vi "CheckStopCondition.vi"(5 "Lower limit":T1={"Fz [pN]"=-100000000.0, "Zext [nm]"=-100000000.0, "Tau [pNnm]"=-100000000.0, "Turn"=-100000000.0, "Fx [pN]"=-100000000.0, "Xext [nm]"=-100000000.0, "Fy [pN]"=-100000000.0, "Yext [nm]"=-100000000.0, "time [s]"=-100000000.0, "Delta Z signal"=-100000000.0, "Delta Z bead [nm]"=-100000000.0, "Z bead [nm]"=-100000000.0, "Delta TrapZ [nm]"=-100000000.0, "Delta Xsignal"=0.0, "X bead [nm]"=-100000000.0, "Delta Ysignal"=-100000000.0, "Y bead [nm]"=-100000000.0, "Stop Condition"=0.0}, 6 "Data":T1, 7 "Upper limit":T1={"Fz [pN]"=100000000.0, "Zext [nm]"=100000000.0, "Tau [pNnm]"=100000000.0, "Turn"=100000000.0, "Fx [pN]"=100000000.0, "Xext [nm]"=100000000.0, "Fy [pN]"=100000000.0, "Yext [nm]"=100000000.0, "time [s]"=100000000.0, "Delta Z signal"=100000000.0, "Delta Z bead [nm]"=100000000.0, "Z bead [nm]"=100000000.0, "Delta TrapZ [nm]"=100000000.0, "Delta Xsignal"=100000000.0, "X bead [nm]"=100000000.0, "Delta Ysignal"=100000000.0, "Y bead [nm]"=100000000.0, "Stop Condition"=100000000.0}) -> (1 "In range?":bool, 2 "Which Signal is out of Range?":u32, 3 "Data out":T1)   [LabVIEW 2020, in "SignalConverson.lvlib"]
uses:
  SignalConverson.lvlib
  Initialization/Physical Quantitites.ctl
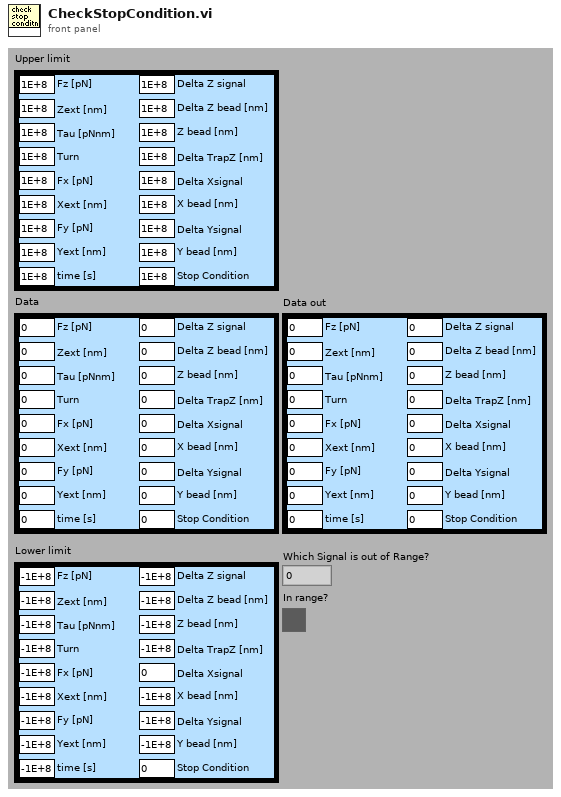
[diagram p1: front panel]
types:
  T1 = typedef "SignalConverson.lvlib/Physical Quantitites.ctl" = cluster{"Fz [pN]":dbl, "Zext [nm]":dbl, "Tau [pNnm]":dbl, "Turn":dbl, "Fx [pN]":dbl, "Xext [nm]":dbl, "Fy [pN]":dbl, "Yext [nm]":dbl, "time [s]":dbl, "Delta Z signal":dbl, "Delta Z bead [nm]":dbl, "Z bead [nm]":dbl, "Delta TrapZ [nm]":dbl, "Delta Xsignal":dbl, "X bead [nm]":dbl, "Delta Ysignal":dbl, "Y bead [nm]":dbl, "Stop Condition":dbl}
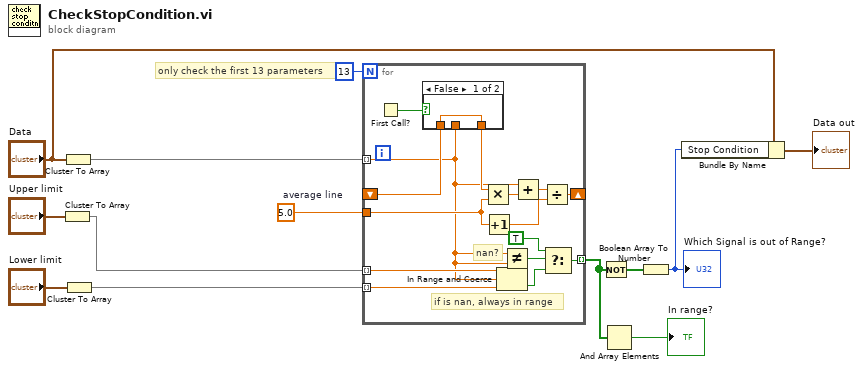
[diagram p0: block diagram]
diagram:
  w6 = 5.0  # average line
  # "only check the first 13 parameters"
  n1 = Cluster To Array(cluster="Upper limit") -> (array=w12:dbl[])
  n2 = Cluster To Array(cluster="Data") -> (array=w10:dbl[])
  n3 = Cluster To Array(cluster="Lower limit") -> (array=w11:dbl[])
  n4 = for {
    N: 13 -> [_]
    tunnel: w12 -> [w28] mode=indexing
    tunnel: w11 -> [w27] mode=indexing
    tunnel: w10 -> [w18] mode=indexing
    tunnel: [w16] -> w8 mode=indexing
    shift-right: [w24] -> _
    shift-left: _ -> [w20]
    tunnel: w6 -> [w22]
    # "if is nan, always in range"
    # "nan?"
    n5 = First Call?() -> (First Call?: T/F=w21:bool)
    n6 = case shown="False" w21 {
      tunnel: w20 -> [w29 _]
      tunnel: [w29 w30] -> w19
      tunnel: w18 -> [_ w30]
      frame False {
      }
      frame True {
      }
    }
    n7 = Multiply(x=w19, y=w22) -> (x*y=w26:dbl)
    n8 = Increment(x=w22) -> (x+1=w23:dbl)
    n9 = In Range and Coerce(upper limit=w28, x=w18, lower limit=w27) -> (In Range?=w15:bool)  [unwired: 1 out]
    n10 = Not Equal?(x=w18, y=w18) -> (x != y?=w17:bool)
    n11 = Add(x=w18, y=w26) -> (x+y=w25:dbl)
    n12 = Divide(x=w25, y=w23) -> (x/y=w24:dbl)
    n13 = Select(t=TRUE, s=w17, f=w15) -> (s? t:f=w16:bool)
  }
  n14 = Not(x=w8) -> (.not. x?=w7:bool[])
  n15 = And Array Elements(Boolean array=w8) -> (logical AND=→"In range?":bool)
  n16 = Boolean Array To Number(Boolean array=w7) -> (number=w5:u32)
  "Which Signal is out of Range?" <- w5
  n17 = Bundle By Name(cluster="Data", "Stop Condition"=w5) -> (→"Data out":T1)
